vi "zigzag.vi"(8 "points":cluster{"x":dbl, "y":dbl}[](array[cluster])=[{"x"=0.0, "y"=0.0}, {"x"=1000.0, "y"=1000.0}], 10 "Current Robot":T1, 11 "Al Input":T3) -> (3 "Output Robot":T1)   [LabVIEW 2016]
uses:
  Core/AI Input.ctl
  Core/AI Robot.ctl
  Intel/Functions Enum.ctl
  Core/AI Ball.ctl
  Core/Field Size.ctl
  Core/AI Judge.ctl
  Intel/Command Enum.ctl
panel:
  out "element 2":cluster{"x":dbl, "y":dbl}
  in  "square tolerance":dbl format="%#_13g"
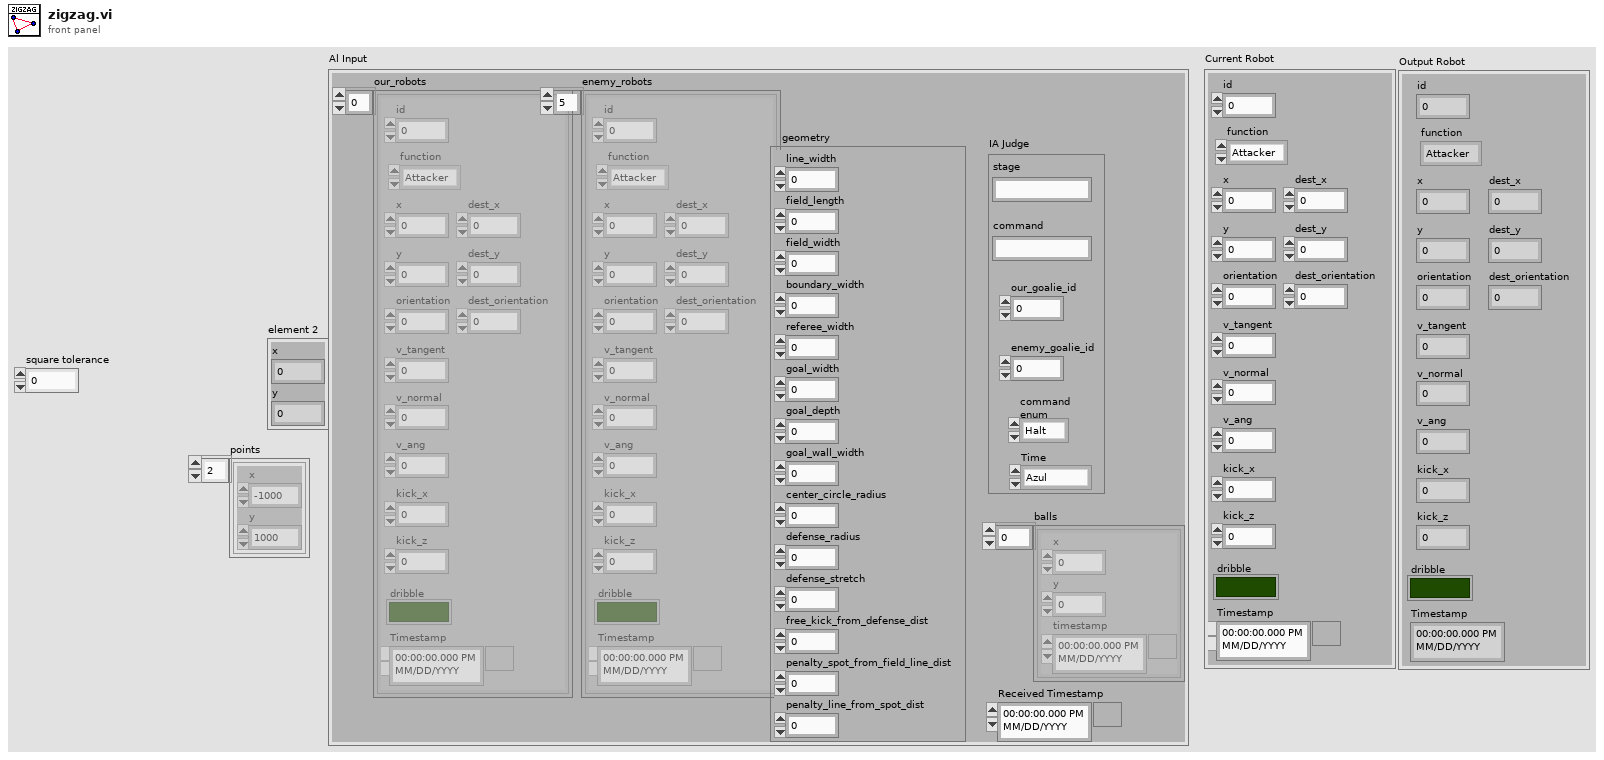
[diagram p1: front panel]
types:
  T1 = typedef "AI Robot.ctl" = cluster{"id":u32, "function":T2, "x":dbl, "y":dbl, "orientation":dbl, "v_tangent":dbl, "v_normal":dbl, "v_ang":dbl, "kick_x":dbl, "kick_z":dbl, "dribble":bool, "Timestamp":timestamp, "dest_x":dbl, "dest_y":dbl, "dest_orientation":dbl}
  T2 = typedef "Functions Enum.ctl" = enum16{"Attacker", "Goalie", "Defender", "Goto 0", "Dummy", "ZigZag"}
  T3 = typedef "AI Input.ctl" = cluster{"our_robots":T1[], "enemy_robots":T1[], "balls":T4[], "geometry":T5, "IA Judge":T6, "Received Timestamp":timestamp}
  T4 = typedef "AI Ball.ctl" = cluster{"x":dbl, "y":dbl, "timestamp":timestamp}
  T5 = typedef "Field Size.ctl" = cluster{"line_width":u32, "field_length":u32, "field_width":u32, "boundary_width":u32, "referee_width":u32, "goal_width":u32, "goal_depth":u32, "goal_wall_width":u32, "center_circle_radius":u32, "defense_radius":u32, "defense_stretch":u32, "free_kick_from_defense_dist":u32, "penalty_spot_from_field_line_dist":u32, "penalty_line_from_spot_dist":u32}
  T6 = typedef "AI Judge.ctl" = cluster{"stage":string, "command":string, "our_goalie_id":dbl, "enemy_goalie_id":dbl, "command\nenum":T7, "Time":enum16{"Azul", "Amarelo"}}
  T7 = typedef "Command Enum.ctl" = enum16{"Halt", "Stop", "Force Start", "PKA Normal Start", "Prepare Kickoff Ally", "PKE Normal Start", "Prepare Kickoff Enemy", "Prepare Penalty Ally", "PPA Normal Start", "Prepare Penalty Enemy", "PPE Normal Start", "Direct Free Enemy", "Direct Free Ally", "Indirect Free Enemy", "Indirect Free Ally", "Timeout Enemy", "Timeout Ally", "Goal Enemy", "Goal Ally", "Ball Placement Enemy", "Ball Placement Ally", "None"}
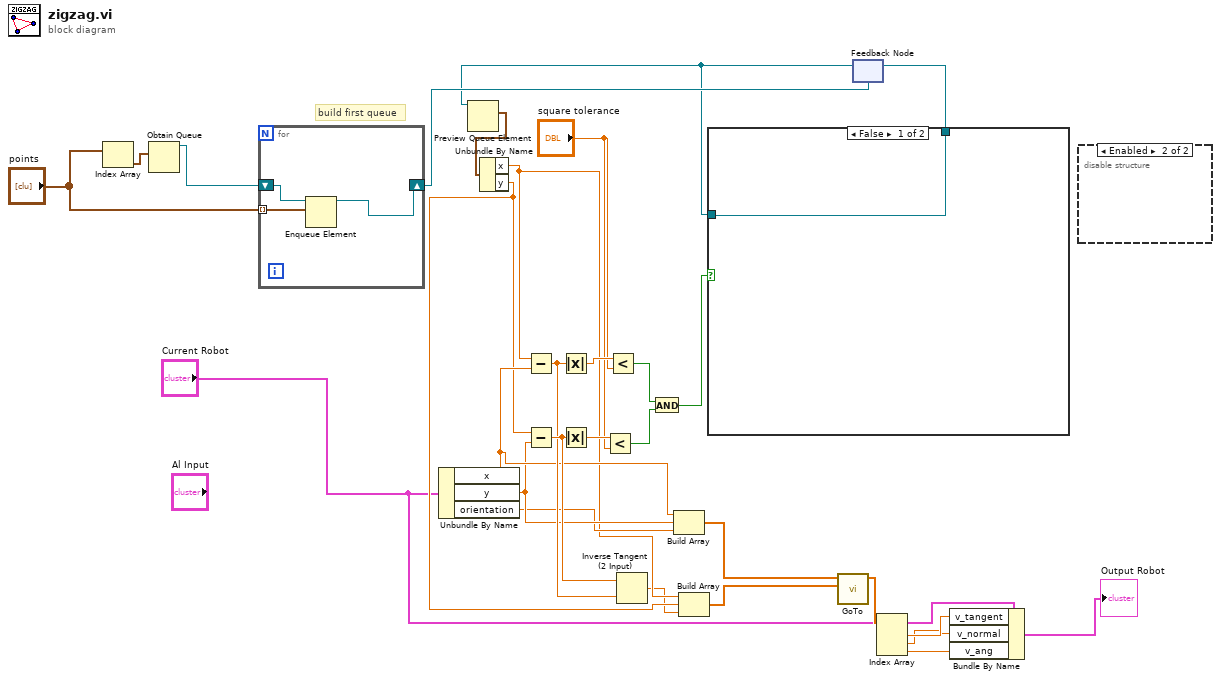
[diagram p0: block diagram]
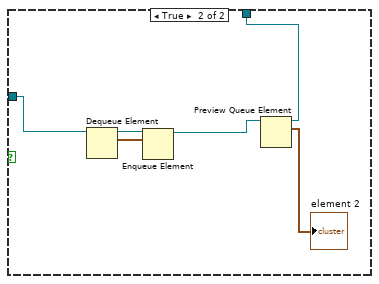
[diagram p2: hidden frame]
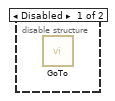
[diagram p3: hidden frame]
diagram:
  # "build first queue"
  n1 = Index Array(array="points") -> (element=w29:cluster{"x":dbl, "y":dbl})  [unwired: 1 in]
  n2 = Obtain Queue(element data type=w29) -> (queue out=w27:refnum<queue>)  [unwired: 4 in, 2 out]
  n3 = for {
    tunnel: "points" -> [w31] mode=indexing
    shift-right: [w32] -> w19
    shift-left: w27 -> [w30]
    n4 = Enqueue Element(queue=w30, element=w31) -> (queue out=w32:refnum<queue>)  [unwired: 2 in, 2 out]
  }
  n5 = Unbundle By Name("Current Robot") -> ("x"=w15:dbl, "y"=w14:dbl, "orientation"=w13:dbl)
  n6 = Build Array(w15, w14, w13) -> (w8:dbl[])
  n7 = feedback #1(w19) -> (w18:refnum<queue>)
  n8 = Preview Queue Element(queue=w18) -> (element=w26:cluster{"x":dbl, "y":dbl})  [unwired: 2 in, 3 out]
  n9 = Unbundle By Name(w26) -> ("x"=w12:dbl, "y"=w11:dbl)
  n10 = Subtract(x=w12, y=w15) -> (x-y=w16:dbl)
  n11 = Subtract(x=w11, y=w14) -> (x-y=w17:dbl)
  n12 = Absolute Value(x=w16) -> (abs(x)=w25:dbl)
  n13 = Absolute Value(x=w17) -> (abs(x)=w24:dbl)
  n14 = Less?(x=w24, y="square tolerance") -> (x < y?=w21:bool)
  n15 = Less?(x=w25, y="square tolerance") -> (x < y?=w22:bool)
  n16 = Inverse Tangent (2 Input)(1:w16, 2:w17) -> (0:w10:dbl)
  n17 = And(x=w22, y=w21) -> (x .and. y?=w20:bool)
  n18 = Build Array(w12, w11, w10) -> (w9:dbl[])
  n19 = case shown="False" w20 {
    tunnel: w18 -> [w33 w37]
    tunnel: [w33 w34] -> w1
    frame False {
    }
    frame True {
      n20 = Dequeue Element(queue=w37) -> (queue out=w38:refnum<queue>, element=w39:cluster{"x":dbl, "y":dbl})  [unwired: 2 in, 2 out]
      n21 = Enqueue Element(queue=w38, element=w39) -> (queue out=w36:refnum<queue>)  [unwired: 2 in, 2 out]
      n22 = Preview Queue Element(queue=w36) -> (queue out=w34:refnum<queue>, element=→"element 2":cluster{"x":dbl, "y":dbl})  [unwired: 2 in, 2 out]
    }
  }
  n23 = call "GoTo.vi"("Target"=w9, "Position"=w8) -> ("Output\nVelocity"=w7:dbl[])  [unwired: 9 in]
  n24 = feedback-in #1(w1) -> ()
  n25 = Index Array(array=w7) -> (element #1=w5:dbl, element #2=w4:dbl, element #3=w3:dbl)  [unwired: 3 in]
  n26 = Bundle By Name(cluster="Current Robot", "v_tangent"=w5, "v_normal"=w4, "v_ang"=w3) -> (→"Output Robot":T1)
  n27 = disable-structure shown="Enabled" {
    frame Disabled {
      n28 = call "GoTo.vi"() -> ()  [unwired: 11 in, 1 out]
    }
    frame Enabled {
    }
  }
